vi "setEventId.vi"(8 "error in (no error)":errorcluster, 10 "eventId":dbl, 11 "SingleToneRamp in":refnum<class "SingleToneRamp.lvclass">) -> (0 "error out":errorcluster, 3 "SingleToneRamp out":refnum<class "SingleToneRamp.lvclass">)   [LabVIEW 2009, in "Tools.lvlib" / "Scripting.lvlib" / "SingleToneRamp.lvclass"]
uses:
  SingleToneRamp.lvclass
  SingleTone.lvclass
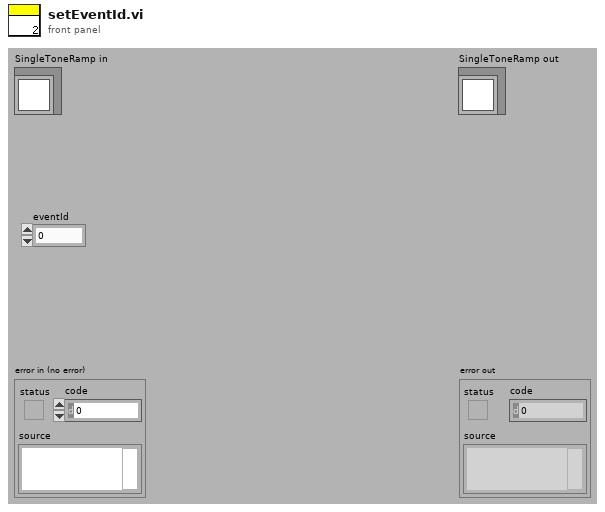
[diagram p1: front panel]
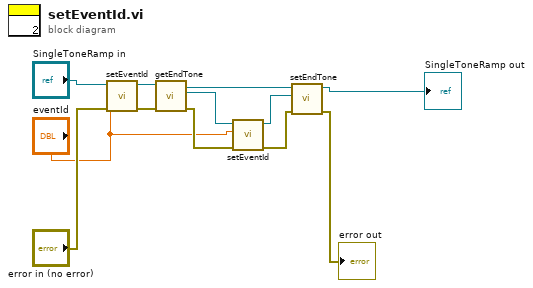
[diagram p0: block diagram]
diagram:
  n1 = call-parent "setEventId.vi"("error in (no error)"="error in (no error)", "eventId"="eventId", "ScriptEvent in"="SingleToneRamp in") -> ("error out"=w3:errorcluster, "ScriptEvent out"=w4:refnum<class "SingleToneRamp.lvclass">)  [unwired: 7 in]
  n2 = call "getEndTone.vi"("error in (no error)"=w3, "SingleToneRamp.lvclass in"=w4) -> ("error out"=w7:errorcluster, "endTone"=w9:refnum<class "SingleTone.lvclass">, "SingleToneRamp.lvclass out"=w10:refnum<class "SingleToneRamp.lvclass">)  [unwired: 7 in]
  n3 = call-parent "setEventId.vi"("error in (no error)"=w7, "eventId"="eventId", "ScriptEvent in"=w9) -> ("error out"=w6:errorcluster, "ScriptEvent out"=w8:refnum<class "SingleTone.lvclass">)  [unwired: 7 in]
  n4 = call "setEndTone.vi"("error in (no error)"=w6, "EndTone"=w8, "SingleToneRamp.lvclass in"=w10) -> ("error out"=→"error out":errorcluster, "SingleToneRamp.lvclass out"=→"SingleToneRamp out":refnum<class "SingleToneRamp.lvclass">)  [unwired: 7 in]
